vi "nimcDMControlLoop_PID(FixedPoint).vi"(1 "PID Gains":T1={"Kp"=50, "Kd"=1000, "Ki"=0, "ILim"=1000, "Kv"=0, "Vff"=0, "Aff"=0, "Td"=0}, 6 "Setpoint":i32, 7 "Commanded Velocity":i32, 8 "Position Feedback":i32, 9 "Commanded Acceleration":i32, 10 "Velocity Feedback":i32, 12 "Position Error Limit":i16=10000) -> (14 "Output":i16, 15 "Position Error Read":i16, 16 "Position Error Status":bool)   [LabVIEW 2014]
doc: "PID Controller - This is a fixed point PID with derivative, integral, velocity feedback, velocity feedforward and acceleration feedforward filtering"
uses:
  <vilib>/rvi/Emulation/niFpgaCriticalErrorInLSC.vi
  <vilib>/rvi/Emulation/niFpgaEmulationReportErrorSimple.vi
  <vilib>/rvi/Emulation/niFpgaSctlEmulationGetInTimedLoop.vi
  <vilib>/rvi/Emulation/niFpgaGetClockAttributes.vi
panel:
  # "Control Loop Output"
  # "Control Loop  Parameters"
  # "Kp - Position gain\nKd - Derivative gain\nKi - Integral gain\nILim - Integral gain limit\nKv - velocity feedback gain\nVff - velocity feedforward gain\nAff - acceleration feedforward gain\nTd - derivative sample period"
  # "Velocity, Commanded Velocity, Commanded Acceleration are in 16.16 format\n- velocity - position increments/control loop period\n- acceleration - position increments/control loop period ^2"
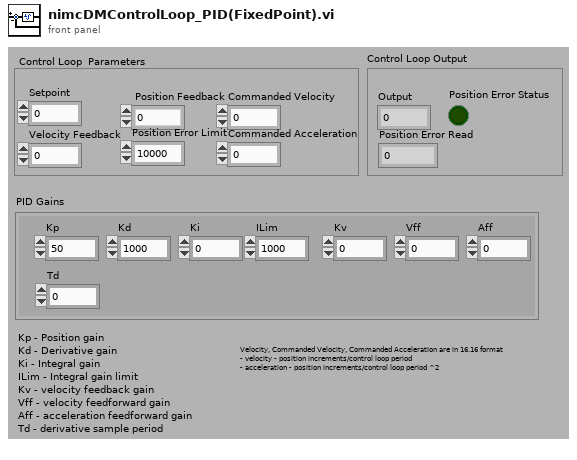
[diagram p1: front panel]
types:
  T1 = cluster{"Kp":i16, "Kd":i16, "Ki":i16, "ILim":i16, "Kv":i16, "Vff":i16, "Aff":i16, "Td":i16}
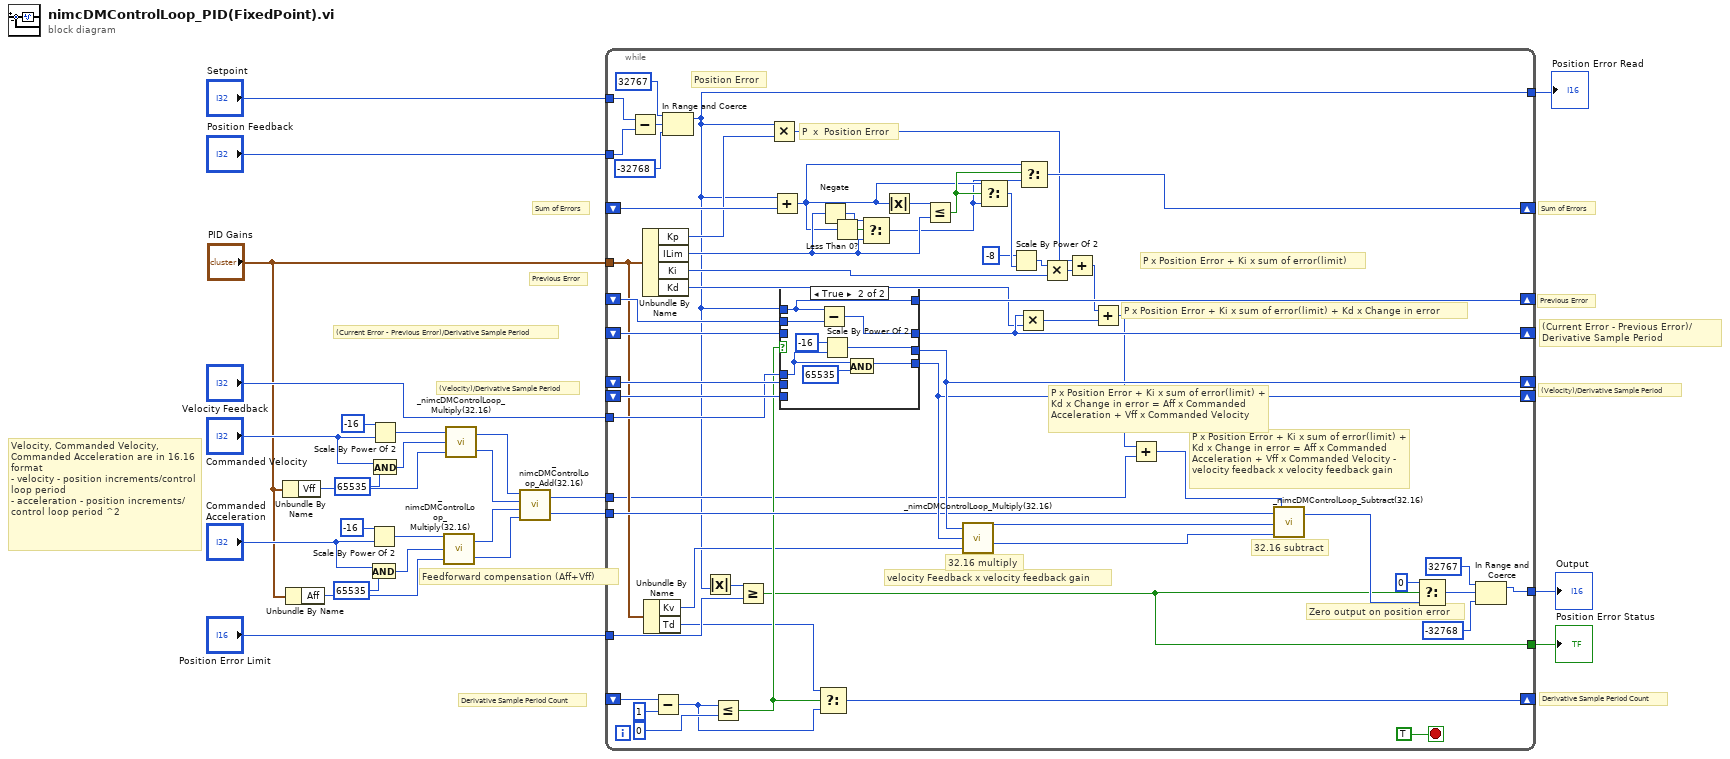
[diagram p0: block diagram]
diagram:
  # "Derivative Sample Period Count"
  # "Derivative Sample Period Count"
  # "(Velocity)/Derivative Sample Period"
  # "Sum of Errors"
  # "Previous Error"
  # "(Current Error - Previous Error)/Derivative Sample Period"
  # "Velocity, Commanded Velocity, Commanded Acceleration are in 16.16 format\n- velocity - position increments/control loop period\n- acceleration - position increments/control loop period ^2"
  # "Feedforward compensation (Aff+Vff)"
  # "(Velocity)/Derivative Sample Period"
  # "(Current Error - Previous Error)/Derivative Sample Period"
  # "Previous Error"
  # "Sum of Errors"
  n1 = Unbundle By Name("PID Gains") -> ("Vff"=w3:i16)
  n2 = Unbundle By Name("PID Gains") -> ("Aff"=w2:i16)
  n3 = Scale By Power Of 2(n=i16 -16, x="Commanded Acceleration") -> (x*2^n=w15:i32)
  n4 = And(x="Commanded Acceleration", y=u32 65535) -> (x .and. y?=w14:u32)
  n5 = Scale By Power Of 2(n=i16 -16, x="Commanded Velocity") -> (x*2^n=w22:i32)
  n6 = And(x="Commanded Velocity", y=u32 65535) -> (x .and. y?=w19:u32)
  n7 = call "_nimcDMControlLoop_Multiply(32.16).vi"("Gain"=w2, "Fraction"=w14, "Integer"=w15) -> ("Fraction"=w10:u16, "Integer"=w11:i32)
  n8 = call "_nimcDMControlLoop_Multiply(32.16).vi"("Gain"=w3, "Fraction"=w19, "Integer"=w22) -> ("Fraction"=w12:u16, "Integer"=w13:i32)
  n9 = call "_nimcDMControlLoop_Add(32.16).vi"("Fraction B"=w10, "Integer B"=w11, "Fraction A"=w12, "Integer A"=w13) -> ("Fraction C"=w8:i16, "Integer C"=w9:i32)
  n10 = while {
    tunnel: "Setpoint" -> [w48]
    tunnel: "Position Feedback" -> [w47]
    tunnel: [w32] -> w26
    shift-left: _ -> [w82]
    shift-right: [w76] -> _
    shift-left: _ -> [w80]
    shift-right: [w49] -> _
    shift-right: [w64] -> _
    shift-left: _ -> [w81]
    shift-right: [w75] -> _
    shift-left: _ -> [w77]
    shift-right: [w74] -> _
    shift-left: _ -> [w69]
    tunnel: w9 -> [w39]
    tunnel: w8 -> [w67]
    tunnel: [w34] -> w7
    tunnel: [w52] -> w6
    tunnel: "Velocity Feedback" -> [w66]
    tunnel: "Position Error Limit" -> [w65]
    tunnel: "PID Gains" -> [w46]
    shift-right: [w54] -> _
    shift-left: _ -> [w58]
    stop <- TRUE stop-if-true
    # "P x Position Error + Ki x sum of error(limit) + Kd x Change in error = Aff x Commanded Acceleration + Vff x Commanded Velocity - velocity feedback x velocity feedback gain"
    # "velocity Feedback x velocity feedback gain"
    # "P x Position Error + Ki x sum of error(limit) + Kd x Change in error = Aff x Commanded Acceleration + Vff x Commanded Velocity"
    # "P x Position Error + Ki x sum of error(limit) + Kd x Change in error"
    # "P x Position Error + Ki x sum of error(limit)"
    # "Zero output on position error"
    # "32.16 subtract"
    # "32.16 multiply"
    # "P  x  Position Error"
    # "Position Error"
    n11 = Subtract(x=w48, y=w47) -> (x-y=w37:i32)
    n12 = Unbundle By Name(w46) -> ("Kp"=w62:i16, "ILim"=w60:i16, "Ki"=w61:i16, "Kd"=w59:i16)
    n13 = Unbundle By Name(w46) -> ("Kv"=w45:i16, "Td"=w38:i16)
    n14 = Subtract(x=w58, y=i16 1) -> (x-y=w55:i16)
    n15 = In Range and Coerce(upper limit=32767, x=w37, lower limit=-32768 ("upper limit")) -> (coerced(x)=w34:i32)  [unwired: 1 out]
    n16 = Absolute Value(x=w34) -> (abs(x)=w83:i32)
    n17 = Less Or Equal?(x=w55, y=i16 0) -> (x <= y?=w53:bool)
    n18 = Greater Or Equal?(x=w83, y=w65) -> (x >= y?=w52:bool)
    n19 = Multiply(x=w34, y=w62) -> (x*y=w44:i32)
    n20 = Add(x=w34, y=w80) -> (x+y=w51:i32)
    n21 = case shown="True" w53 {
      tunnel: [w89 w90] -> w64
      tunnel: w82 -> [w87 w97]
      tunnel: w34 -> [_ w96]
      tunnel: w81 -> [w89 _]
      tunnel: w77 -> [w88 _]
      tunnel: [w88 w91] -> w75
      tunnel: w66 -> [_ w94]
      tunnel: [w87 w96] -> w76
      tunnel: w69 -> [w86 _]
      tunnel: [w86 w92] -> w74
      frame False {
      }
      frame True {
        n22 = Subtract(x=w96, y=w97) -> (x-y=w90:i32)
        n23 = Scale By Power Of 2(n=i16 -16, x=w94) -> (x*2^n=w91:i32)
        n24 = And(x=w94, y=u32 65535) -> (x .and. y?=w92:u32)
      }
    }
    n25 = Select(t=w38, s=w53, f=w55) -> (s? t:f=w54:i16)
    n26 = Negate(x=w60) -> (-x=w70:i16)
    n27 = Less Than 0?(x=w51) -> (x < 0?=w71:bool)
    n28 = Select(t=w70, s=w71, f=w60) -> (s? t:f=w50:i16)
    n29 = Absolute Value(x=w51) -> (abs(x)=w79:i32)
    n30 = Less Or Equal?(x=w79, y=w60) -> (x <= y?=w78:bool)
    n31 = call "_nimcDMControlLoop_Multiply(32.16).vi"("Gain"=w45, "Fraction"=w74, "Integer"=w75) -> ("Fraction"=w72:u16, "Integer"=w73:i32)
    n32 = Select(t=w51, s=w78, f=w50) -> (s? t:f=w29:i32)
    n33 = Scale By Power Of 2(n=-8, x=w29) -> (x*2^n=w27:i32)
    n34 = Multiply(x=w64, y=w59) -> (x*y=w41:i32)
    n35 = Select(t=w51, s=w78, f=w50) -> (s? t:f=w49:i32)
    n36 = Multiply(x=w27, y=w61) -> (x*y=w43:i32)
    n37 = Add(x=w44, y=w43) -> (x+y=w42:i32)
    n38 = Add(x=w42, y=w41) -> (x+y=w40:i32)
    n39 = Add(x=w40, y=w39) -> (x+y=w68:i32)
    n40 = call "_nimcDMControlLoop_Subtract(32.16).vi"("Fraction B"=w72, "Integer B"=w73, "Fraction A"=w67, "Integer A"=w68) -> ("Integer A-B"=w63:i32)  [unwired: 1 out]
    n41 = Select(t=0, s=w52, f=w63) -> (s? t:f=w33:i32)
    n42 = In Range and Coerce(upper limit=32767, x=w33, lower limit=-32768) -> (coerced(x)=w32:i32)  [unwired: 1 out]
  }
  "Output" <- w26
  "Position Error Status" <- w6
  "Position Error Read" <- w7
